vi "PM-A-Acquisition_main_sim.vi"(8 "error in":errorcluster, 11 "init_cluster":T1) -> (0 "error out":errorcluster)   [LabVIEW 2018]
uses:
  init-close/PM-init-data_cluster.ctl
  init-close/PM-init-user_events.ctl
  init-close/PM-common-heartrate_data.ctl
  init-close/PM-common-peak-detect_settings.ctl
  PM-A-aqn_loop_data.ctl
panel:
  in  "aqn?":bool
  in  "Stop":bool
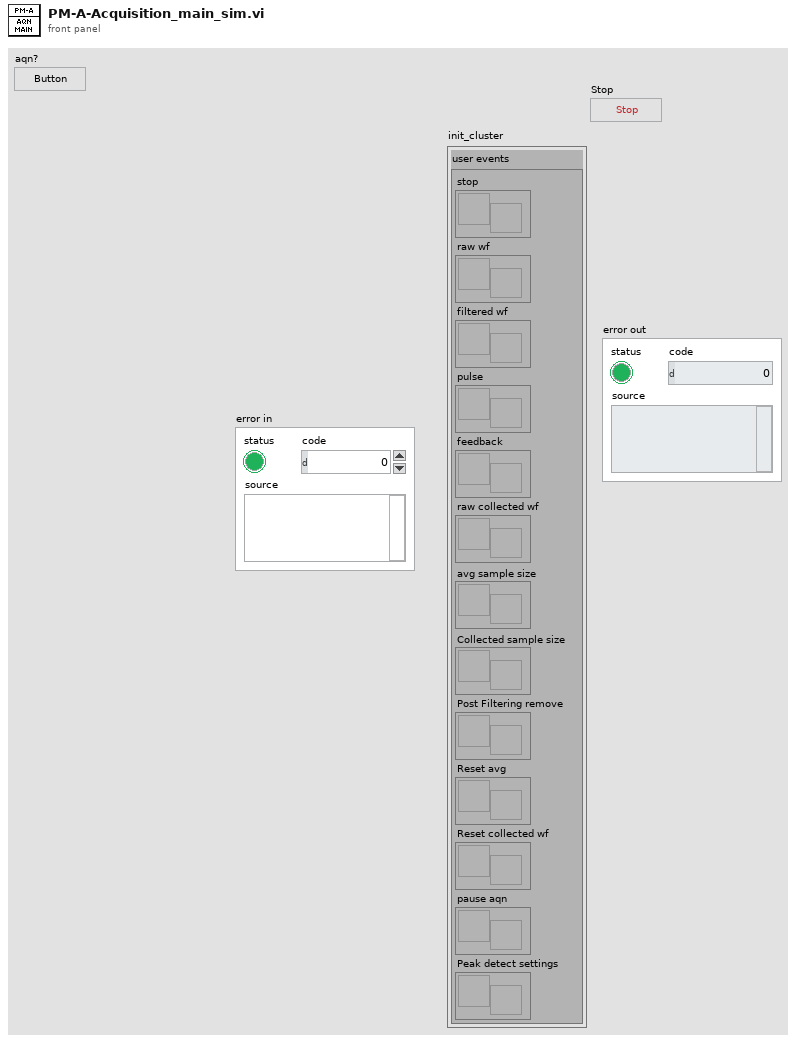
[diagram p1: front panel]
types:
  T1 = typedef "PM-init-data_cluster.ctl" = cluster{"user events":T2}
  T2 = typedef "PM-init-user_events.ctl" = cluster{"stop":refnum<user-event>, "raw wf":refnum<user-event>, "filtered wf":refnum<user-event>, "pulse":refnum<user-event>, "feedback":refnum<user-event>, "raw collected wf":refnum<user-event>, "avg sample size":refnum<user-event>, "Collected sample size":refnum<user-event>, "Post Filtering remove":refnum<user-event>, "Reset avg":refnum<user-event>, "Reset collected wf":refnum<user-event>, "pause aqn":refnum<user-event>, "Peak detect settings":refnum<user-event>}
  T3 = typedef "PM-A-aqn_loop_data.ctl" = cluster{"Stop event":refnum<user-event>, "Raw wf event":refnum<user-event>}
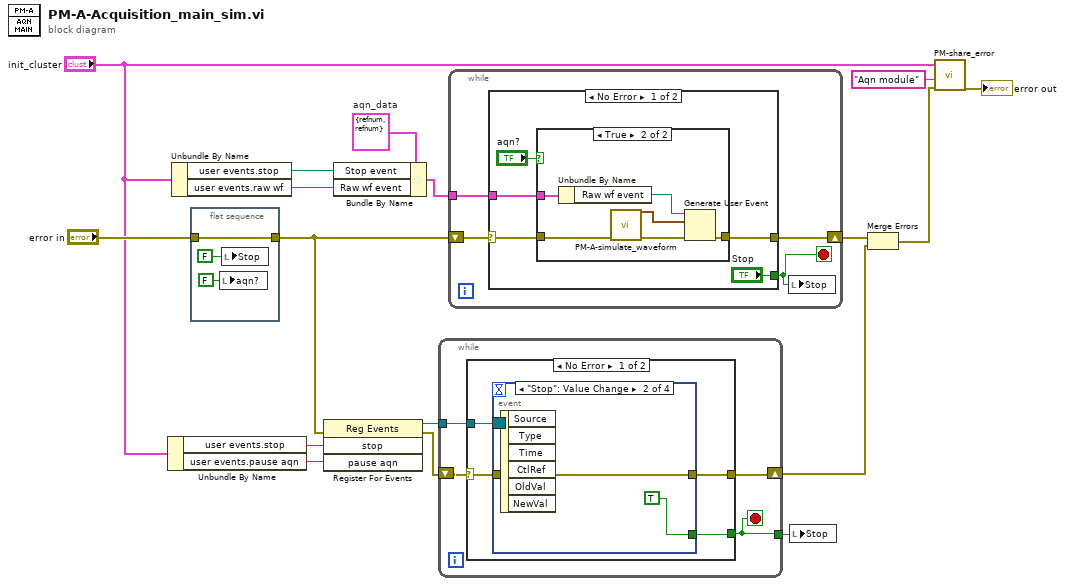
[diagram p0: block diagram]
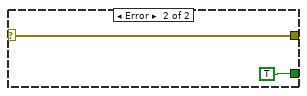
[diagram p3: hidden frame]
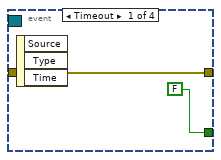
[diagram p4: hidden frame]
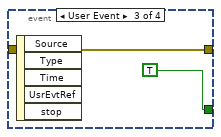
[diagram p5: hidden frame]
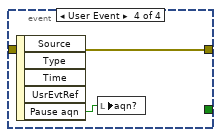
[diagram p6: hidden frame]
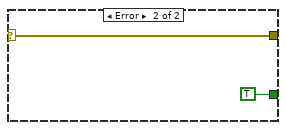
[diagram p7: hidden frame]
diagram:
  w11 = T3 {"Stop event"=refnum, "Raw wf event"=refnum}  # aqn_data
  n1 = Unbundle By Name("init_cluster") -> ("user events.stop"=w13:refnum<user-event>, "user events.pause aqn"=w1:refnum<user-event>)
  n2 = Unbundle By Name("init_cluster") -> ("user events.stop"=w9:refnum<user-event>, "user events.raw wf"=w8:refnum<user-event>)
  n3 = flat-sequence {
    tunnel: "error in" -> [w19]
    tunnel: [w19] -> w6
    frame #0 {
      n4 = local write "aqn?"(FALSE ("aqn?")) -> ()
      n5 = local write "Stop"(FALSE ("Stop")) -> ()
    }
  }
  n6 = register-events(error in=w6, w13, w1) -> (reference out=w12:refnum<event-registration>, error out=w14:errorcluster)  [unwired: 1 in]
  n7 = Bundle By Name(cluster=w11, "Stop event"=w9, "Raw wf event"=w8) -> (w10:T3)
  n8 = while {
    tunnel: [w23] -> w17
    shift-right: [w22] -> w16
    shift-left: w14 -> [w24]
    tunnel: w12 -> [w21]
    stop <- w23 stop-if-true
    n9 = case shown="No Error" w24 {
      selector: w24 -> [w26 w37]
      tunnel: [w28 TRUE] -> w23
      tunnel: [w27 w37] -> w22
      tunnel: w21 -> [w25 _]
      frame No Error {
        n10 = event shown="[1] \"Stop\": Value Change" {
          selector: w25 -> [_ _ _ _]
          dyn-events: _ -> [_ _ _ _]
          timeout: _ -> [_ _ _ _]
          tunnel: [FALSE TRUE TRUE _] -> w28
          tunnel: [w29 w32 w34 w36] -> w27
          tunnel: w26 -> [w29 w32 w34 w36]
          event Timeout {
            n11 = event-data() -> ()  [unwired: 1 in, 3 out]
          }
          event "Stop": Value Change {
            n12 = event-data() -> ()  [unwired: 1 in, 6 out]
          }
          event User Event {
            n13 = event-data() -> ()  [unwired: 1 in, 5 out]
          }
          event User Event {
            n14 = event-data() -> ("Pause aqn"=w35:bool)  [unwired: 1 in, 4 out]
            n15 = local write "aqn?"(w35) -> ()
          }
        }
      }
      frame Error {
      }
    }
  }
  n16 = while {
    shift-right: [w41] -> w15
    shift-left: w6 -> [w42]
    tunnel: w10 -> [w39]
    stop <- w40 stop-if-true
    n17 = case shown="No Error" w42 {
      selector: w42 -> [w46 w56]
      tunnel: ["Stop" TRUE ("Stop")] -> w40
      tunnel: [w45 w56] -> w41
      tunnel: w39 -> [w44 _]
      frame No Error {
        n18 = case shown="True" "aqn?" {
          tunnel: w46 -> [w48 w54]
          tunnel: [w48 w53] -> w45
          tunnel: w44 -> [_ w52]
          frame False {
          }
          frame True {
            n19 = Unbundle By Name(w52) -> ("Raw wf event"=w51:refnum<user-event>)
            n20 = call "PM-A-simulate_waveform.vi"("error in (no error)"=w54) -> ("error out"=w49:errorcluster, "signal out"=w50:waveform(dbl))  [unwired: 9 in]
            n21 = Generate User Event(user event=w51, event data cluster=w50, error in=w49) -> (error out=w53:errorcluster)  [unwired: 1 in, 1 out]
          }
        }
      }
      frame Error {
      }
    }
    n22 = local write "Stop"(w40) -> ()
  }
  n23 = local write "Stop"(w17) -> ()
  n24 = Merge Errors(w15, w16) -> (w5:errorcluster)
  n25 = call "PM-share_error.vi"("error in (no error)"=w5, "module name"="Aqn module", "init_cluster"="init_cluster") -> ("error out"=→"error out":errorcluster)  [unwired: 8 in]
